vi "turn on off LED.vi"() -> ()   [LabVIEW 2015]
uses:
  <vilib>/MakerHub/LINX/Public/Peripherals/Digital/Digital Write 1 Chan.vi
  <vilib>/MakerHub/LINX/Public/Peripherals/Digital/Digital Write N Chans.vi
  <vilib>/MakerHub/LINX/Private/Local IO/LinxDigitalWrite.vi
  <vilib>/MakerHub/LINX/Public/Utilities/Check Channel.vi
  <vilib>/MakerHub/LINX/Public/Utilities/Open Serial.vi
  <vilib>/MakerHub/LINX/Private/Utilties/Generate Error.vi
  <vilib>/MakerHub/LINX/LMH-LINX.lvlib
panel:
  in  "AO Channel":u8
  in  "Boolean":bool
  in  "stop":bool
  in  "Serial Port":refnum<visa-resource-name>="N/A"
  out "Loop Rate (Hz)":u32
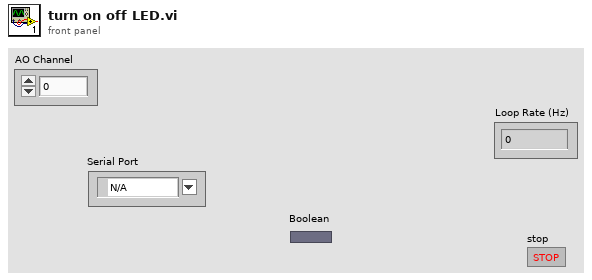
[diagram p1: front panel]
types:
  T1 = typedef "LMH-LINX.lvlib/LINX Ref.ctl" = cluster{"IO":T2, "Interface":T3, "LINX Device Config":T4}
  T2 = typedef "LMH-LINX.lvlib/Platform.ctl" = enum16{"Remote", "Local"}
  T3 = typedef "LMH-LINX.lvlib/Interface.ctl" = enum16{"Serial", "TCP"}
  T4 = typedef "LMH-LINX.lvlib/Device.lvlib/LINX Device Config.ctl" = cluster{"Interface":T3, "COM Port":refnum<visa-resource-name>, "TCP Configuration":T5, "Device Family":u8, "Device ID":u8, "Device Name":string, "TCP Ref":refnum<k5>, "Channels":T6}
  T5 = typedef "LMH-LINX.lvlib/Device.lvlib/TCP Config.ctl" = cluster{"IP Address":string, "Port":u16}
  T6 = typedef "LMH-LINX.lvlib/Channels.ctl" = cluster{"DI":u8[], "DO":u8[], "AI":u8[], "AO":u8[], "PWM":u8[], "QE":u8[], "UART":u8[], "I2C 2":u8[], "SPI":u8[], "CAN":u8[], "Servo":u8[], "AI Ref (V)":dbl, "AI Resolution (Bits)":u8, "AO Ref (V)":dbl, "AO Resolution (Bits)":u8}
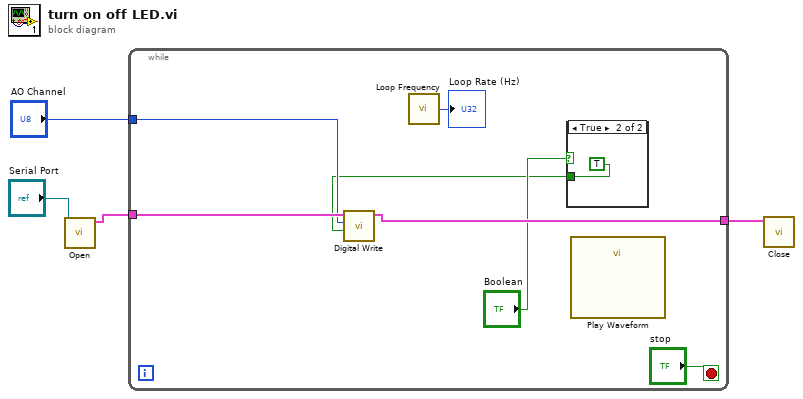
[diagram p0: block diagram]
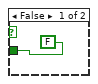
[diagram p2: hidden frame]
diagram:
  n1 = call-poly <vilib>:"Open.vi"("Serial Port"="Serial Port") -> ("LINX Resource"=w3:T1)  [unwired: 8 in, 2 out]
  n2 = while {
    tunnel: w3 -> [w10]
    tunnel: [w9] -> w2
    tunnel: "AO Channel" -> [w6]
    stop <- "stop" stop-if-true
    n3 = call <vilib>:"Loop Frequency.vi"() -> ("Loop Rate (Hz)"=→"Loop Rate (Hz)":u32)
    n4 = case shown="True" "Boolean" {
      tunnel: [FALSE TRUE] -> w5
      frame False {
      }
      frame True {
      }
    }
    n5 = call-poly <vilib>:"Digital Write.vi"("Output Value"=w5, "DO Channel"=w6, "LINX Resource"=w10) -> ("LINX Resource"=w9:T1)  [unwired: 7 in, 1 out]
    n6 = call "Play Waveform"() -> ()  [unwired: 19 in, 1 out]
  }
  n7 = call <vilib>:"Close.vi"("LINX Resource"=w2) -> ()  [unwired: 10 in, 1 out]
